vi "F Dwf Analog Out Repeat Get.vi"(8 "error in (no error)":errorcluster, 9 "pcRepeat":i32, 10 "idxChannel":i32, 11 "hdwf":i32) -> (0 "error out":errorcluster, 1 "pcRepeat out":i32, 3 "function return":i32)   [LabVIEW 2019, in "Olasdwf.lvlib"]
doc: "DWFAPI int FDwfAnalogOutRepeatGet(HDWF hdwf, int idxChannel, int *pcRepeat);"
uses:
  Olasdwf.lvlib
  Windows/System32/dwf.dll
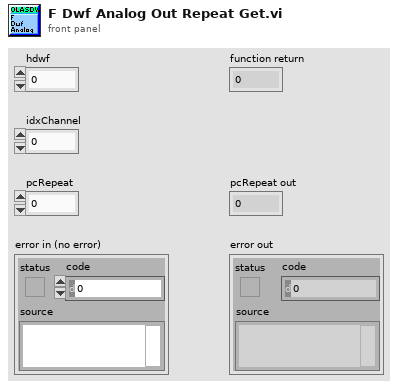
[diagram p1: front panel]
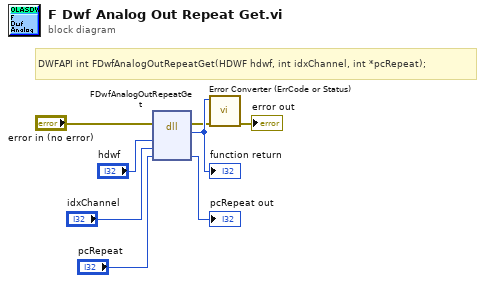
[diagram p0: block diagram]
diagram:
  # "DWFAPI int FDwfAnalogOutRepeatGet(HDWF hdwf, int idxChannel, int *pcRepeat);"
  n1 = dll-call lib="C:/Windows/System32/dwf.*" fn="FDwfAnalogOutRepeatGet"(error in="error in (no error)", "hdwf"="hdwf", "idxChannel"="idxChannel", "pcRepeat"="pcRepeat") -> (error out=w2:errorcluster, w8:i32, "pcRepeat"=→"pcRepeat out":i32)  [unwired: 4 in, 1 out]
  "function return" <- w8
  n2 = call "Error Converter (ErrCode or Status).vi"("error in (no error)"=w2, "error code"=w8) -> ("error out"=→"error out":errorcluster)  [unwired: 9 in]
